vi "Program list Selection.vi"(8 "error in":errorcluster, 9 "FeedBack Channel":string[](array[string])=["fgdgfvcbc", "vnfhgjkn", "21354682"], 10 "Filepath":path=path "D:/My Project/2019-2020/Magnetic Mareli UM/MM_UM/Project Setup/data/program seq/Program_280A.bin", 11 "vi referenceIn":refnum<vi>) -> (0 "error out":errorcluster, 1 "Exit":bool, 2 "String":string, 3 "vi reference Out":refnum<vi>)   [LabVIEW 2015]
uses:
  Control Button/Exit.ctl
  Control Button/next.ctl
  Galobal variable_TI.vi
  <vilib>/addons/database/Connection.llb/DB Tools Open Connec (String).vi
  <vilib>/addons/database/_DB Variant To Data/Database Variant To Data.xnode
  <vilib>/addons/database/NI_Database_API.lvlib
panel:
  out "error out 2":errorcluster
  in  "Cluster 3":T1
  out "error out 3":errorcluster
  out "String 2":string
  in  "Next":T2
  in  "Exit":T3
  in  "Program List":string(combo)
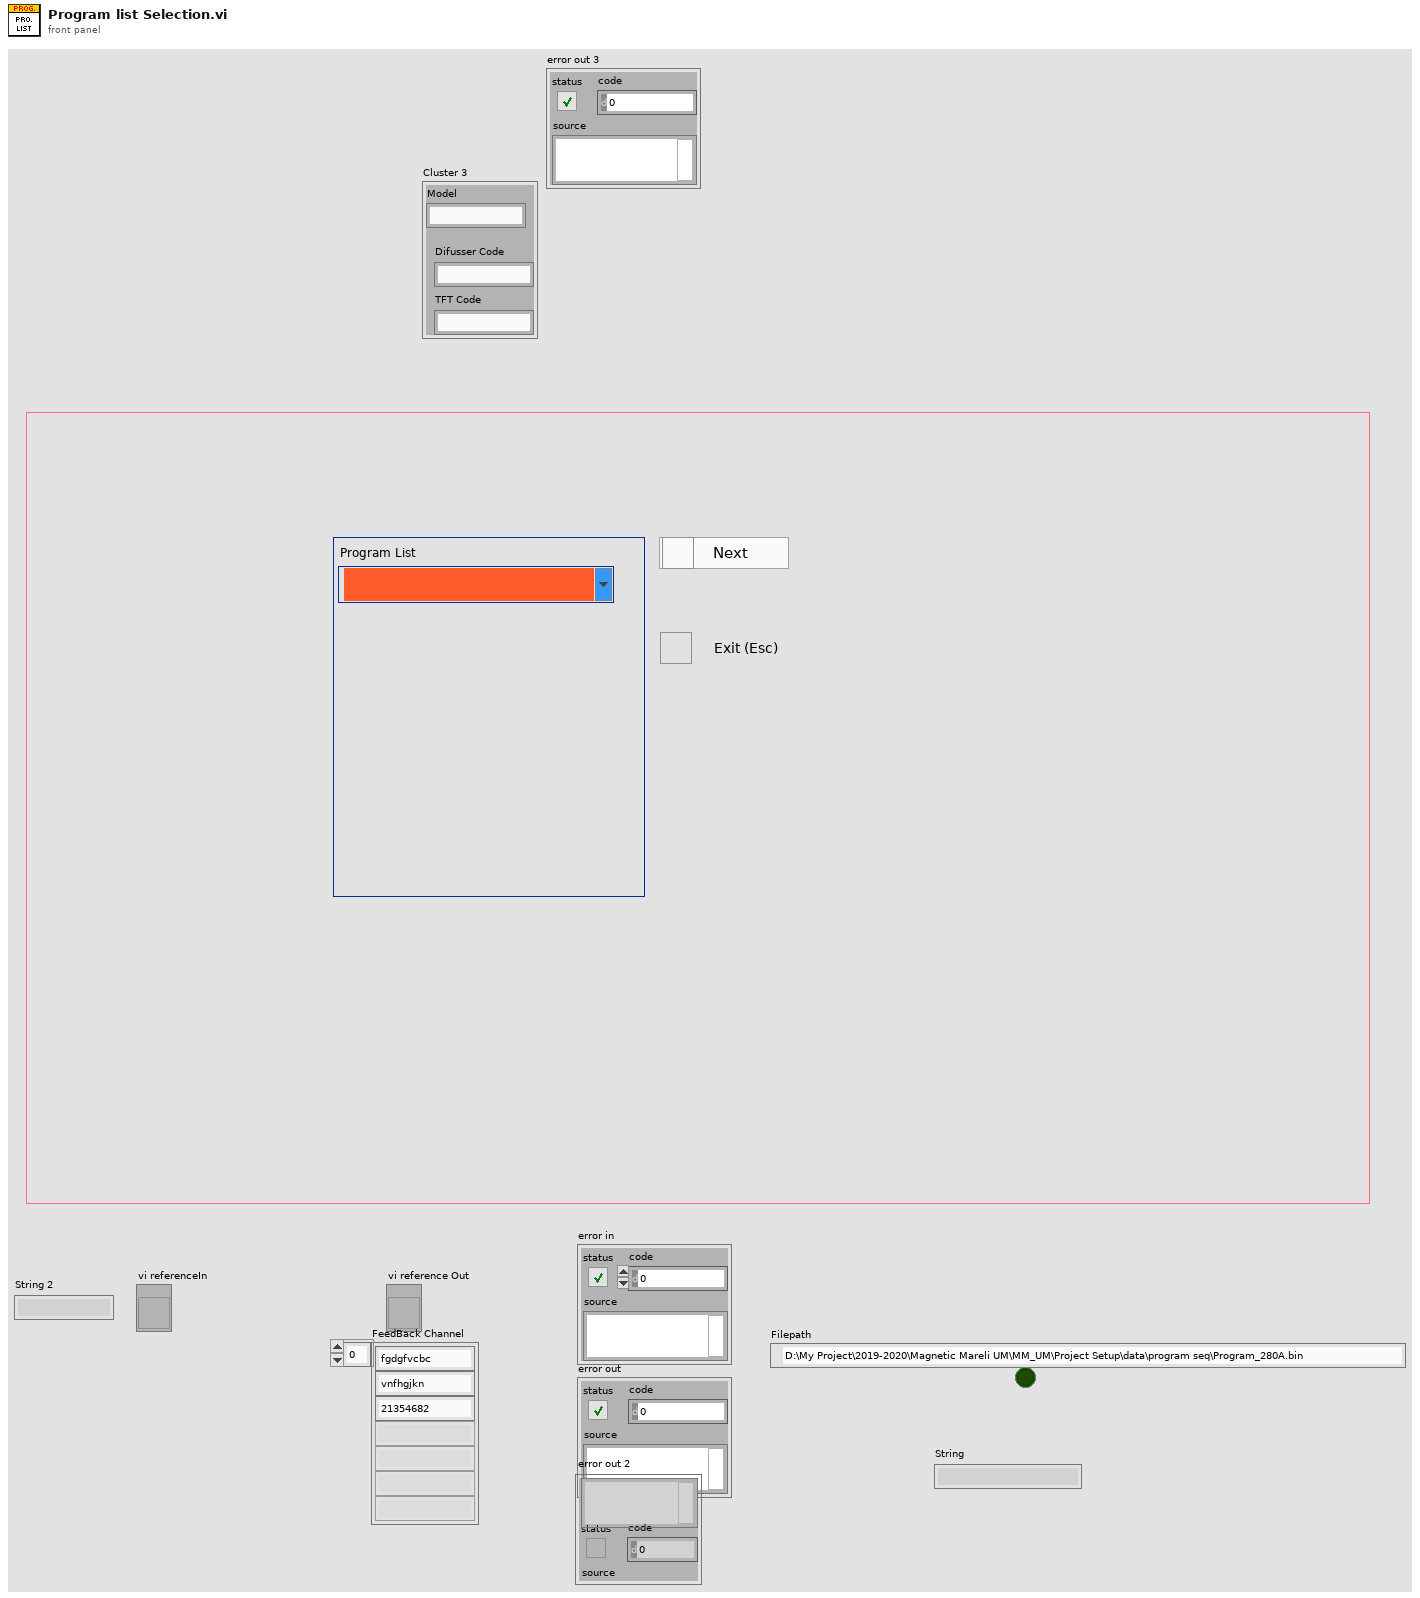
[diagram p1: front panel]
types:
  T1 = cluster{"Model":string, "Difusser Code":string, "TFT Code ":string}
  T2 = typedef "next.ctl" = bool
  T3 = typedef "Exit.ctl" = bool
  T4 = enum32{"Invalid", "Standard", "Closed", "Hidden", "Minimized", "Maximized"}
  T5 = typedef "NI_Database_API.lvlib/Conn ObjectReference.ctl" = refnum<k1>
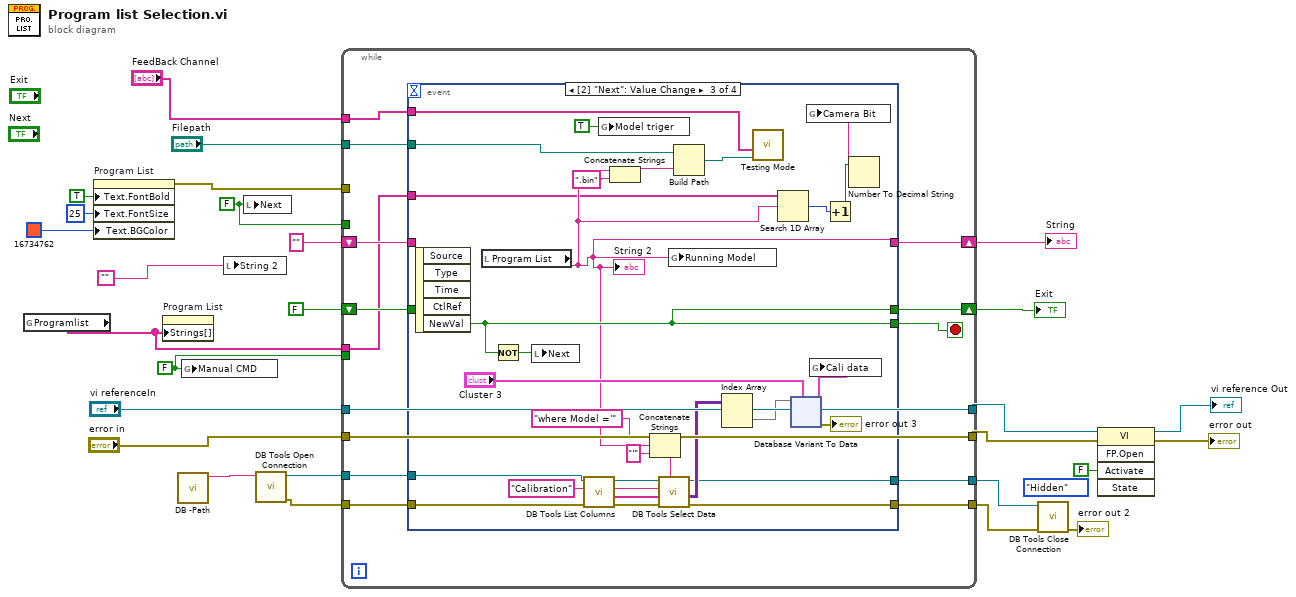
[diagram p0: block diagram]
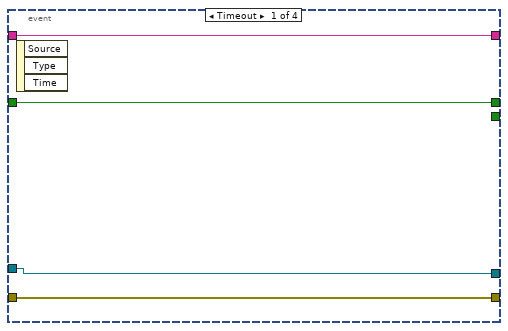
[diagram p2: hidden frame]
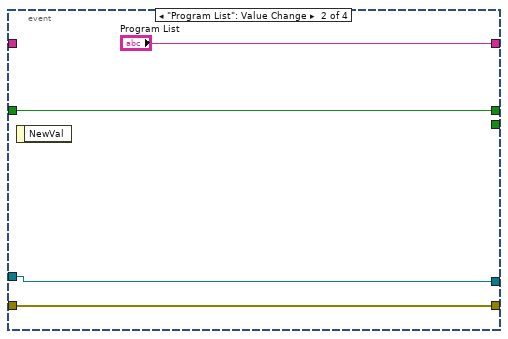
[diagram p3: hidden frame]
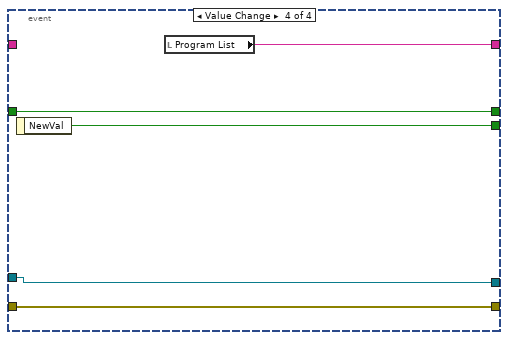
[diagram p4: hidden frame]
diagram:
  (unwired) T4."Hidden" ("State")
  w16 = FALSE ("Manual CMD")
  w17 = FALSE ("Next")
  n1 = global read "Galobal variable_TI.vi" "Programlist"() -> (w23:string[])
  n2 = property on="Program List" class="CmbBox"("Text.FontBold"=TRUE ("Text.Font:Bold"), "Text.FontSize"=u32 25 ("Text.Font:Size"), "Text.BGColor"=u32 16734762 ("Color Box")) -> (error out=w20:errorcluster)  [unwired: 2 in, 1 out]
  n3 = property on="Program List" class="CmbBox"("Strings[]"=w23) -> ()  [unwired: 2 in, 2 out]
  n4 = call "DB -Path.vi"() -> ("String"=w4:string)  [unwired: 11 in]
  n5 = global write "Galobal variable_TI.vi" "Manual CMD"(w16) -> ()
  n6 = local write "String 2"("") -> ()
  n7 = local write "Next"(w17) -> ()
  n8 = call-poly <vilib>:"DB Tools Open Connection.vi"("connection information"=w4) -> ("error out"=w5:errorcluster, "connection reference"=w6:T5)  [unwired: 7 in]
  n9 = while {
    shift-right: [w41] -> w27
    shift-left: "" ("Combo Box") -> [w40]
    shift-right: [w38] -> w24
    shift-left: T3 FALSE ("NewVal") -> [w37]
    tunnel: w23 -> [w30]
    tunnel: w20 -> [_]
    tunnel: w17 -> [_]
    tunnel: w16 -> [_]
    tunnel: "vi referenceIn" -> [w36]
    tunnel: [w36] -> w10
    tunnel: "error in" -> [w35]
    tunnel: [w35] -> w9
    tunnel: "Filepath" -> [w34]
    tunnel: "FeedBack Channel" -> [w33]
    tunnel: w6 -> [w32]
    tunnel: w5 -> [w31]
    tunnel: [w29] -> w3
    tunnel: [w28] -> w2
    stop <- w39 stop-if-true
    n10 = event shown="[2] \"Next\": Value Change" {
      selector: _ -> [_ _ _ _]
      dyn-events: _ -> [_ _ _ _]
      timeout: _ -> [_ _ _ _]
      tunnel: [w45 "Program List" w57 w179] -> w41
      tunnel: w40 -> [w45 _ _ _]
      tunnel: [_ _ w73 w180] -> w39
      tunnel: [w44 w48 w73 w178] -> w38
      tunnel: w37 -> [w44 w48 _ w178]
      tunnel: w34 -> [_ _ w76 _]
      tunnel: w33 -> [_ _ w74 _]
      tunnel: w32 -> [w43 w47 w60 w177]
      tunnel: w31 -> [w42 w46 w59 w176]
      tunnel: w30 -> [_ _ w53 _]
      tunnel: [w43 w47 w51 w177] -> w29
      tunnel: [w42 w46 w50 w176] -> w28
      event Timeout {
        n11 = event-data() -> ()  [unwired: 1 in, 3 out]
      }
      event "Program List": Value Change {
        n12 = event-data() -> ()  [unwired: 1 in, 1 out]
      }
      event Value Change {
        w64 = "Calibration" ("table")
        n13 = event-data() -> ("NewVal"=w73:T2)  [unwired: 1 in, 4 out]
        n14 = local read "Program List"() -> (w57:string)
        "String 2" <- w57
        n15 = Not(x=w73) -> (.not. x?=w72:T2)
        n16 = local write "Next"(w72) -> ()
        n17 = call <vilib>:"DB Tools List Columns.vi"("error in (no error)"=w59, "table"=w64, "connection reference"=w60) -> ("error out"=w67:errorcluster, "columns"=w65:string[], "connection reference out"=w66:T5)  [unwired: 1 in, 1 out]
        n18 = global write "Galobal variable_TI.vi" "Model triger"(TRUE ("Model triger")) -> ()
        n19 = Concatenate Strings(w57, ".bin" ("string")) -> (w77:string)
        n20 = Concatenate Strings("where Model ='" ("string"), w57, "'" ("string")) -> (w68:string)
        n21 = call <vilib>:"DB Tools Select Data.vi"("condition"=w68, "error in (no error)"=w67, "columns"=w65, "table"=w64, "connection reference"=w66) -> ("error out"=w50:errorcluster, "data"=w69:variant[][], "connection reference out"=w51:T5)  [unwired: 1 in]
        n22 = global write "Galobal variable_TI.vi" "Running Model"(w57) -> ()
        n23 = Build Path(base path=w76, name or relative path=w77) -> (appended path=w75:path)
        n24 = Index Array(array=w69) -> (element=w61:variant[])  [unwired: 2 in]
        n25 = call "Testing Mode.vi"("Filepath"=w75, "FeedBack Channel"=w74) -> ()  [unwired: 10 in]
        n26 = Search 1D Array(1D array=w53, element=w57) -> (index of element=w56:i32)  [unwired: 1 in]
        n27 = xnode "Database Variant To Data"("database variant"=w61, "type"="Cluster 3") -> ("data"=w58:T1, "error out"=→"error out 3":errorcluster)  [unwired: 1 in]
        n28 = global write "Galobal variable_TI.vi" "Cali data"(w58) -> ()
        n29 = Increment(x=w56) -> (x+1=w55:i32)
        n30 = Number To Decimal String(number=w55) -> (decimal integer string=w54:string)  [unwired: 1 in]
        n31 = global write "Galobal variable_TI.vi" "Camera Bit"(w54) -> ()
      }
      event Value Change {
        n32 = event-data() -> ("NewVal"=w180:T3)  [unwired: 1 in]
        n33 = local read "Program List"() -> (w179:string)
      }
    }
  }
  "String" <- w27
  "Exit" <- w24
  n34 = call <vilib>:"DB Tools Close Connection.vi"("error in (no error)"=w2, "connection reference"=w3) -> ("error out"=→"error out 2":errorcluster)  [unwired: 5 in]
  n35 = invoke class="VI" method="FP.Open"(reference=w10, error in=w9, "Activate"=FALSE ("Activate?")) -> (reference out=→"vi reference Out":refnum<vi>, error out=→"error out":errorcluster)  [unwired: 2 in, 3 out]
